vi "Get Symbols.vi"(8 "error in (no error)":errorcluster, 10 "Project Path":path, 11 "App Instance":refnum<vi>) -> (0 "error out":errorcluster, 2 "Symbols":map{string, string}(c390))   [LabVIEW 2020, in "Conditional Disabled Configurator.lvclass"]
uses:
  Conditional Disabled Configurator.lvclass
  Conditional Disabled Configurator.lvclass/Conditional Disabled Configurator.ctl
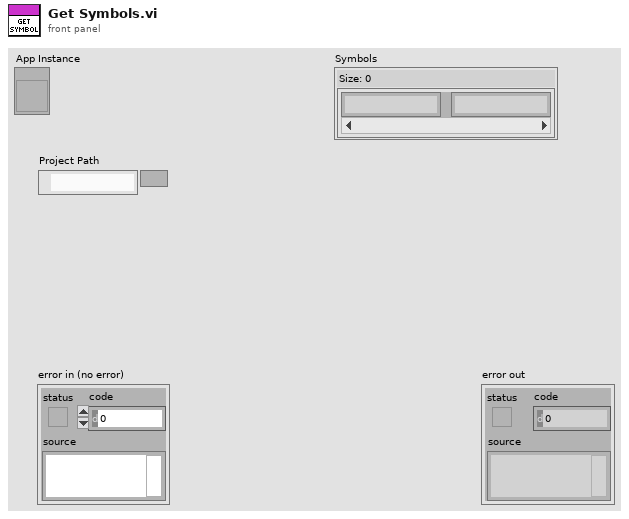
[diagram p1: front panel]
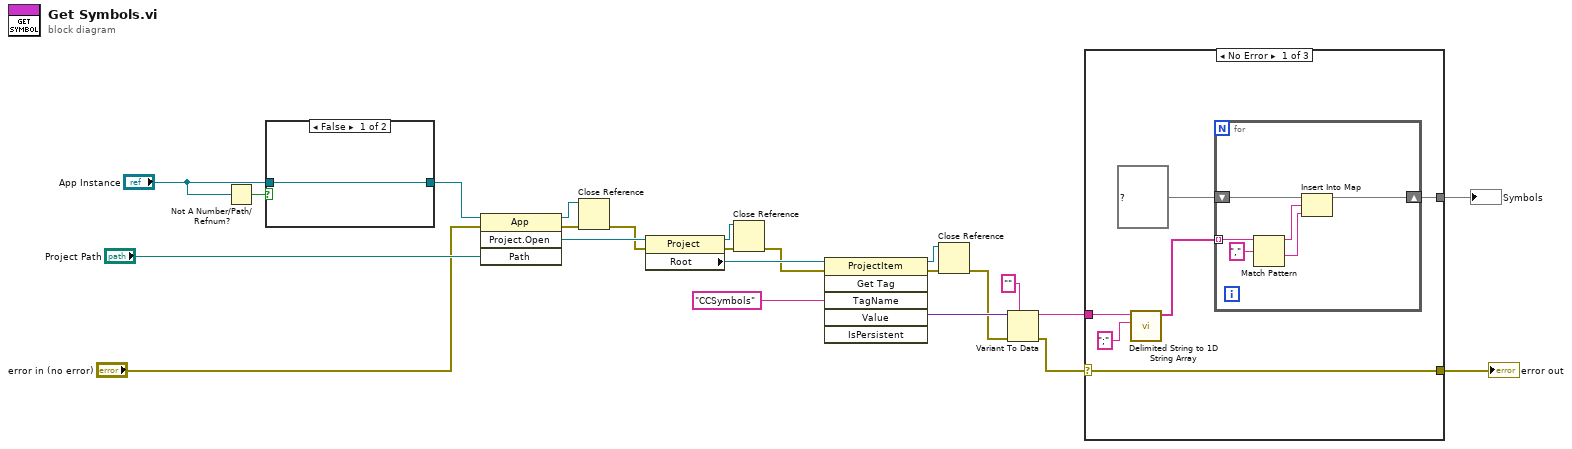
[diagram p0: block diagram]
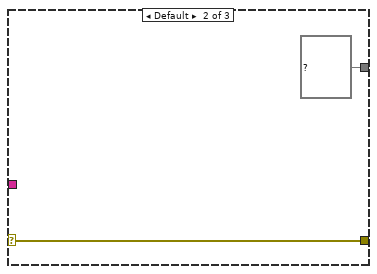
[diagram p2: hidden frame]
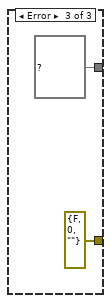
[diagram p3: hidden frame]
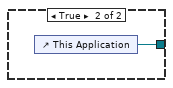
[diagram p4: hidden frame]
diagram:
  n1 = Not A Number/Path/Refnum?(number/path/refnum="App Instance") -> (NaN/Path/Refnum?=w11:bool)
  n2 = case shown="False" w11 {
    tunnel: [w24 w25] -> w10
    tunnel: "App Instance" -> [w24 _]
    frame False {
    }
    frame True {
      n3 = control-ref of="This Application"() -> (w25:refnum<vi>)
    }
  }
  n4 = invoke class="App" method="Project.Open"(reference=w10, error in="error in (no error)", "Path"="Project Path") -> (reference out=w5:refnum<vi>, error out=w20:errorcluster, "Project:Open"=w23:refnum<vi>)  [unwired: 1 in, 1 out]
  n5 = Close Reference(reference=w5, error in (no error)=w20) -> (error out=w6:errorcluster)
  n6 = property class="Project"(reference=w23, error in=w6) -> (reference out=w3:refnum<vi>, error out=w18:errorcluster, "Root"=w22:refnum<vi>)
  n7 = Close Reference(reference=w3, error in (no error)=w18) -> (error out=w4:errorcluster)
  n8 = invoke class="ProjectItem" method="Get Tag"(reference=w22, error in=w4, "TagName"="CCSymbols" ("Tag Name")) -> (reference out=w1:refnum<vi>, error out=w15:errorcluster, "Value"=w16:variant)  [unwired: 3 in, 3 out]
  n9 = Close Reference(reference=w1, error in (no error)=w15) -> (error out=w2:errorcluster)
  n10 = Variant To Data(error in=w2, type="", Variant=w16) -> (data=w14:string, error out=w8:errorcluster)
  n11 = case shown="No Error" w8 {
    selector: w8 -> [w26 w39 _]
    tunnel: w14 -> [w31 _ _]
    tunnel: [w28 map{string, string} {} ("Symbols") map{string, string} {} ("Symbols")] -> w12
    tunnel: [w26 w39 errorcluster {"status"=FALSE, "code"=0, "source"=""} ("error IO")] -> w7
    frame No Error {
      n12 = call <vilib>:"Delimited String to 1D String Array.vi"("delimiter"=";", "delimited string"=w31) -> ("string array"=w27:string[])  [unwired: 9 in]
      n13 = for {
        shift-right: [w36] -> w28
        shift-left: map{string, string} {} ("Symbols") -> [w37]
        tunnel: w27 -> [w35] mode=indexing
        n14 = Match Pattern(string=w35, regular expression=",") -> (before substring=w33:string, after substring=w32:string)  [unwired: 1 in, 2 out]
        n15 = Insert Into Map(map in=w37, key=w33, value=w32) -> (map out=w36:map{string, string})  [unwired: 2 out]
      }
    }
    frame Default {
    }
    frame Error {
    }
  }
  "error out" <- w7
  "Symbols" <- w12
